vi "Scan Engine Rename Slot.vi"(8 "error in (no error)":errorcluster, 9 "Name reference":refnum<vi>, 10 "Module Model":T2, 11 "Node Ptr In":T1 format="%.0x") -> (0 "error out":errorcluster, 3 "Node Ptr Out":T1 format="%.0x")   [LabVIEW 2016, in "Scan Engine Custom Device.lvlib"]
uses:
  Scan Engine Custom Device.lvlib
  <vilib>/NI Veristand/Custom Device API/Custom Device API.lvlib
  Globals/Scan Engine GUIDs.vi
  Modules.lvlibp/RSI Module/Module Models.ctl
  <vilib>/NI Veristand/Custom Device API/Custom Device Item Ref.ctl
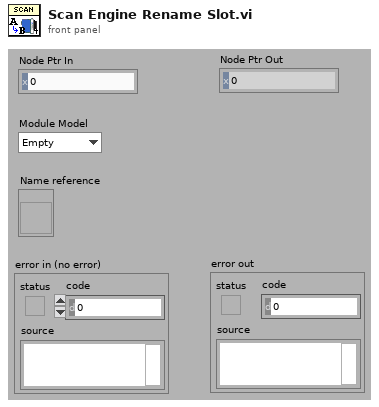
[diagram p1: front panel]
types:
  T1 = typedef "Custom Device API.lvlib/Custom Device Item Ref.ctl" = u64
  T2 = typedef "Modules.lvlibp/RSI Module.lvclass/Module Models.ctl" = enum16{"Empty", "NI 9201", "NI 9203", "NI 9205", "NI 9206", "NI 9207", "NI 9208", "NI 9211", "NI 9213", "NI 9214", "NI 9215", "NI 9217", "NI 9219", "NI 9221", "NI 9225", "NI 9227", "NI 9229", "NI 9233", "NI 9234", "NI 9235", "NI 9236", "NI 9237", "NI 9239", "NI 9263", "NI 9264", "NI 9265", "NI 9269", "NI 9375", "NI 9401", "NI 9402", "NI 9403", "NI 9411", "NI 9421", "NI 9422", "NI 9423", "NI 9425", "NI 9426", "NI 9435", "NI 9472", "NI 9474", "NI 9475", "NI 9476", "NI 9477", "NI 9478", "NI 9481", "NI 9482", "NI 9485"}
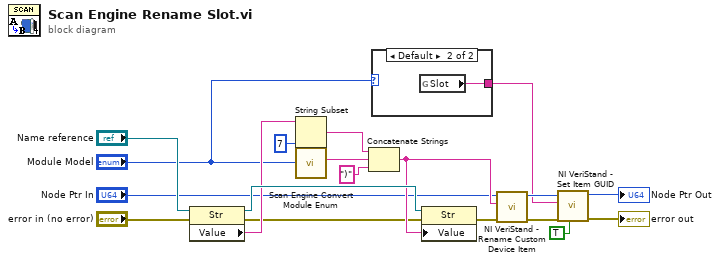
[diagram p0: block diagram]
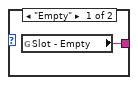
[diagram p2: hidden frame]
diagram:
  n1 = property class="Str"(reference="Name reference", error in="error in (no error)") -> (reference out=w17:refnum<vi>, error out=w9:errorcluster, "Value"=w15:string)
  n2 = String Subset(string=w15, length (rest)=7 ("length (rest)")) -> (substring=w13:string)  [unwired: 1 in]
  n3 = call "Scan Engine Convert Module Enum.vi"("Module"="Module Model") -> ("Module Name"=w19:string)  [unwired: 2 in, 1 out]
  n4 = Concatenate Strings(w13, w19, ")" ("string")) -> (w10:string)
  n5 = case shown="Default" "Module Model" {
    tunnel: [w20 w21] -> w4
    frame "Empty" {
      n6 = global read "Scan Engine GUIDs.vi" "Slot - Empty"() -> (w20:string)
    }
    frame Default {
      n7 = global read "Scan Engine GUIDs.vi" "Slot"() -> (w21:string)
    }
  }
  n8 = property class="Str"(reference=w17, error in=w9, "Value"=w10) -> (error out=w11:errorcluster)  [unwired: 1 out]
  n9 = call <vilib>:"NI VeriStand - Rename Custom Device Item.vi"("error in (no error)"=w11, "New Name"=w10, "Item Ref in"="Node Ptr In") -> ("error out"=w6:errorcluster, "Item Ref out"=w7:T1)  [unwired: 1 in, 6 out]
  n10 = call <vilib>:"NI VeriStand - Set Item GUID.vi"("Refresh System Explorer Tree? (F)"=TRUE, "error in (no error)"=w6, "GUID"=w4, "Item Ref in"=w7) -> ("error out"=→"error out":errorcluster, "Item Ref out"=→"Node Ptr Out":T1)  [unwired: 6 in]
